vi "Install Package.vi"(7 "Logger":refnum<class "Logger.lvclass">, 8 "error in (no error)":errorcluster, 11 "NamedPackage in":refnum<class "NamedPackage.lvclass">) -> (0 "error out":errorcluster, 3 "NamedPackage out":refnum<class "NamedPackage.lvclass">)   [LabVIEW 2020, in "GPack.lvlib" / "NamedPackage.lvclass"]
uses:
  NamedPackage.lvclass
  Logger/Logger.lvclass
  NamedPackage.lvclass/NamedPackage.ctl
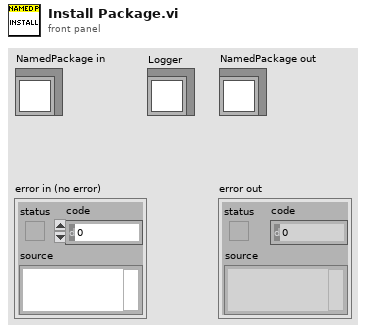
[diagram p1: front panel]
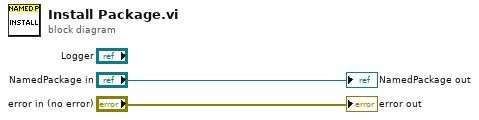
[diagram p0: block diagram]
diagram:
  "error out" <- "error in (no error)"
  "NamedPackage out" <- "NamedPackage in"
